vi "Get Object Pointer.vi"(8 "error in (no error)":errorcluster, 11 "Connection in":refnum<class "Connection.lvclass">) -> (0 "error out":errorcluster, 1 "Assigned object pointer?":bool, 2 "Object Pointer":i64, 3 "Connection out":refnum<class "Connection.lvclass">)   [LabVIEW 2015, in "MDSplus.lvlib" / "Connection.lvclass"]
uses:
  <vilib>/MDSplus/Classes/Connection_Class/Connection.lvclass
  <vilib>/MDSplus/Classes/Connection_Class/Connection.lvclass/Connection.ctl
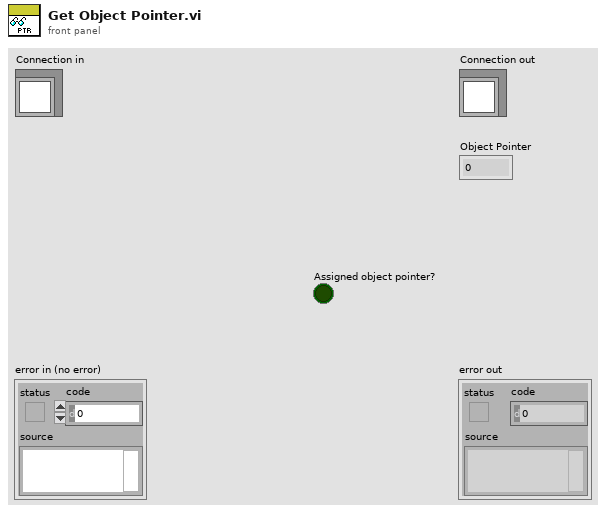
[diagram p1: front panel]
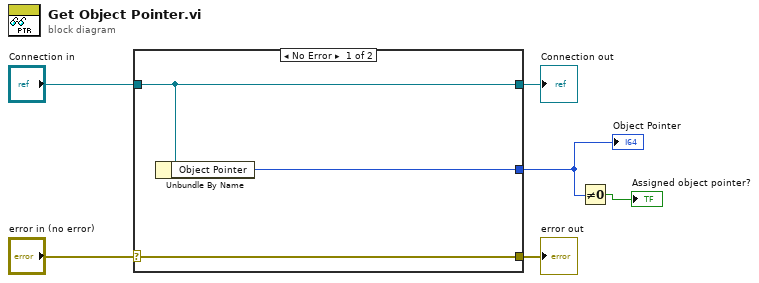
[diagram p0: block diagram]
diagram:
  n1 = case shown="No Error" "error in (no error)" {
    selector: "error in (no error)" -> [w9 w10]
    tunnel: [w9 w10] -> w5
    tunnel: [w8 w11] -> w3
    tunnel: "Connection in" -> [w8 w11]
    tunnel: [w7 _] -> w1
    frame No Error {
      n2 = Unbundle By Name(w8) -> ("Object Pointer"=w7:i64)
    }
    frame Error {
    }
  }
  "error out" <- w5
  "Connection out" <- w3
  "Object Pointer" <- w1
  n3 = Not Equal To 0?(x=w1) -> (x != 0?=→"Assigned object pointer?":bool)
